vi "Setup.vi"(0 "SA Path in":refnum<class "SA Path.lvclass">, 11 "error in (no error)":errorcluster) -> (4 "SA Path out":refnum<class "SA Path.lvclass">, 15 "error out":errorcluster)   [LabVIEW 2023, in "RFFixtureCharact.Public.lvlib" / "SA Path.lvclass"]
uses:
  SA Path.lvclass
  C:/srd-semi-rfcal-software/AuxTools/STSRFFixtureCharactUtility/Source/Code Modules/Common/Base Classes/Path/Path.lvclass
  C:/srd-semi-rfcal-software/AuxTools/STSRFFixtureCharactUtility/Source/Code Modules/Fixture/Public/Base Classes/Scalar/SA Abstract Path/SA Abstract Path.lvclass
  SA Abstract Path/SA Abstract Path.lvclass/SA Abstract Path.ctl
  SA Abstract Path/Properties/Read Cal Tone Pin.vi
  SA Abstract Path/SA Abstract Path.lvclass
  Common/RFCalAndFixtureCharact.Common.lvlib
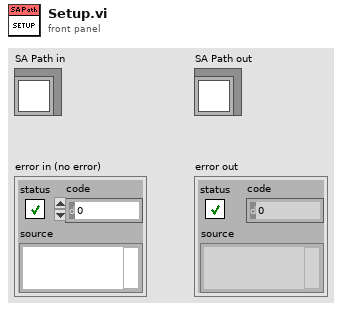
[diagram p1: front panel]
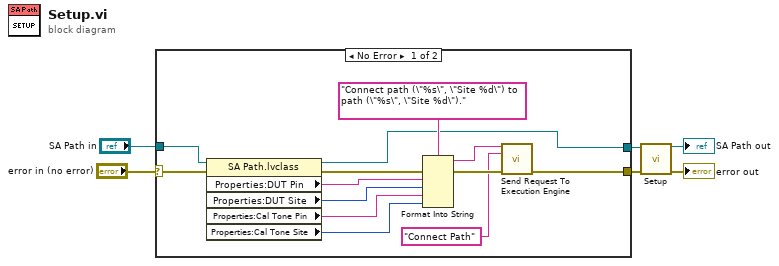
[diagram p0: block diagram]
diagram:
  n1 = case shown="No Error" "error in (no error)" {
    selector: "error in (no error)" -> [w19 w21]
    tunnel: [w11 w20] -> w3
    tunnel: [w12 w21] -> w4
    tunnel: "SA Path in" -> [w10 w20]
    frame No Error {
      n2 = property class="SA Path.lvclass"(reference=w10, error in=w19) -> (reference out=w11:refnum<class "SA Path.lvclass">, error out=w18:errorcluster, "Properties:DUT Pin"=w8:string, "Properties:DUT Site"=w7:i32, "Properties:Cal Tone Pin"=w17:string, "Properties:Cal Tone Site"=w9:i32)
      n3 = Format Into String(format string="Connect path (\"%s\", \"Site %d\") to path (\"%s\", \"Site %d\").", error in=w18, w8, w7, w17, w9) -> (resulting string=w14:string, error out=w15:errorcluster)  [unwired: 1 in]
      n4 = call "Send Request To Execution Engine.vi"("Request Message"=w14, "Request Header"="Connect Path", "error in (no error)"=w15) -> ("error out"=w12:errorcluster)  [unwired: 11 in, 1 out]
    }
    frame Error {
    }
  }
  n5 = call-parent "Setup.vi"("Scalar SA Path in"=w3, "error in (no error)"=w4) -> ("Scalar SA Path out"=→"SA Path out":refnum<class "SA Path.lvclass">, "error out"=→"error out":errorcluster)  [unwired: 12 in]
